vi "Unrecoverable Writer Error.vi"() -> ()   [LabVIEW 2024]
uses:
  Logger/Logger.lvclass
  Handlers/Test Handler/Test Handler.lvclass
  Handlers/File Handler/File Handler.lvclass
  Log Levels.ctl
  Logging.lvlib
  Logger/Internal Log Levels.ctl
  Log Record.ctl
panel:
  out "fail info":T3 {"Log Record"."timestamp" format="%<%x %.3X>T"}
  out "error out":errorcluster
  # "Locals"
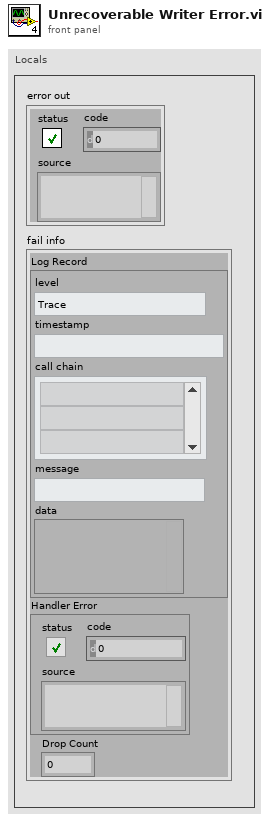
[diagram p1: front panel]
types:
  T1 = typedef "Logging.lvlib/Log Record.ctl" = cluster{"level":T2, "timestamp":timestamp, "call chain":string[], "message":string, "data":variant}
  T2 = typedef "Logging.lvlib/Internal Log Levels.ctl" = enum16{"Trace", "Debug", "Info", "Warning", "Error", "Critical", "Internal"}
  T3 = cluster{"Log Record":T1, "Handler Error":errorcluster, "Drop Count":u32}
  T4 = typedef "Logging.lvlib/Log Levels.ctl" = enum16{"Trace", "Debug", "Info", "Warning", "Error", "Critical"}
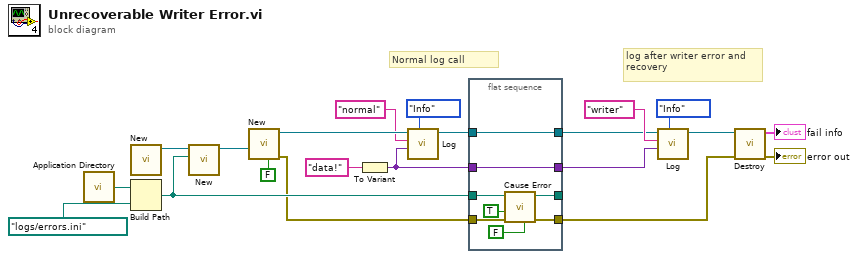
[diagram p0: block diagram]
diagram:
  # "log after writer error and recovery"
  # "Normal log call"
  n1 = call <vilib>:"Application Directory.vi"() -> ("Application Directory"=w7:path)
  n2 = call "New.vi"() -> ("file handler"=w21:refnum<class "File Handler.lvclass">)  [unwired: 11 in]
  n3 = Build Path(base path=w7, name or relative path=path "logs/errors.ini") -> (appended path=w13:path)
  n4 = call "New.vi"("config file"=w13, "subhandler"=w21) -> ("test handler out"=w20:refnum<class "Test Handler.lvclass">)  [unwired: 9 in]
  n5 = call "New.vi"("dialog on failure? (T)"=FALSE, "log handler (file handler)"=w20) -> ("error out"=w12:errorcluster, "logger"=w18:refnum<class "Logger.lvclass">)  [unwired: 8 in]
  n6 = To Variant(anything="data!" ("message")) -> (Variant=w4:variant)
  n7 = call "Log.vi"("log level"=Log_Levels."Info" ("level"), "data (null)"=w4, "message"="normal", "logger in"=w18) -> ("logger out"=w9:refnum<class "Logger.lvclass">)  [unwired: 7 in]
  n8 = flat-sequence {
    tunnel: w13 -> [w29]
    tunnel: w12 -> [w28]
    tunnel: [w27] -> w11
    tunnel: [w26] -> _
    tunnel: [w25] -> w10
    tunnel: w9 -> [w25]
    tunnel: [w24] -> w3
    tunnel: w4 -> [w24]
    frame #0 {
      n9 = call "Cause Error.vi"("writer recovery? (T)"=FALSE, "error in (no error)"=w28, "writer error? (F)"=TRUE ("formatter error? (F)"), "ini file path"=w29) -> ("error out"=w27:errorcluster, "ini file path"=w26:path)  [unwired: 6 in]
    }
  }
  n10 = call "Log.vi"("log level"=Log_Levels."Info" ("level"), "data (null)"=w3, "message"="writer", "logger in"=w10) -> ("logger out"=w8:refnum<class "Logger.lvclass">)  [unwired: 7 in]
  n11 = call "Destroy.vi"("error in (no error)"=w11, "logger in"=w8) -> ("error out"=→"error out":errorcluster, "fail info"=→"fail info":T3)  [unwired: 8 in]
